vi "AH Bridge Read.vi"(6 "Read Frequency":bool, 9 "Boolean":bool, 10 "Average Time (mS)":u32, 11 "Instrument Address":refnum<visa-resource-name>) -> (2 "Measurement":dbl[](array[numeric]) format="%_6e", 3 "dup Instrument Address":refnum<visa-resource-name>)   [LabVIEW 2021]
uses:
  <vilib>/regexp/Match Regular Expression.xnode
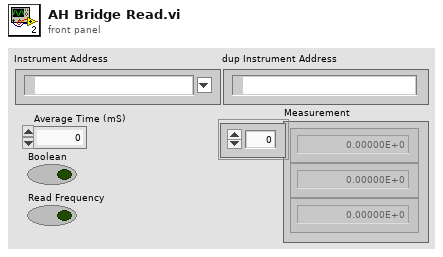
[diagram p1: front panel]
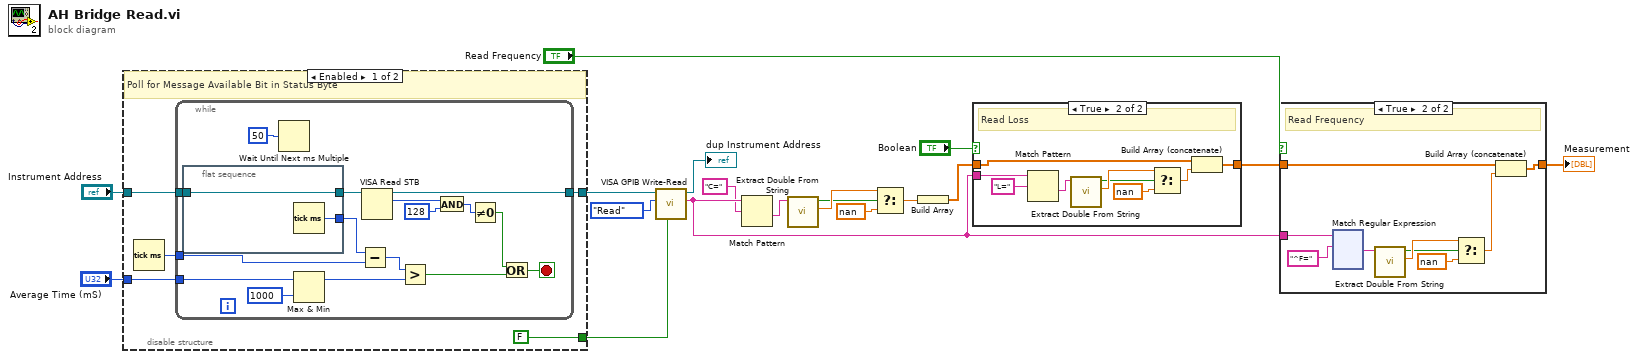
[diagram p0: block diagram]
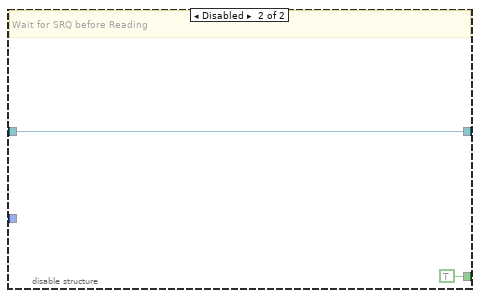
[diagram p2: hidden frame]
diagram:
  n1 = disable-structure shown="Enabled" {
    disable-tunnel: [w23 w43] -> w17
    disable-tunnel: "Instrument Address" -> [w21 w43]
    disable-tunnel: "Average Time (mS)" -> [w20 _]
    disable-tunnel: [FALSE ("Wait For SRQ") TRUE ("Wait For SRQ")] -> w3
    frame Enabled {
      # "Poll for Message Available Bit in Status Byte"
      n2 = Tick Count (ms)() -> (millisecond timer value=w22:u32)
      n3 = while {
        tunnel: [w33] -> w23
        tunnel: w21 -> [w29]
        tunnel: w22 -> [w32]
        tunnel: w20 -> [w27]
        stop <- w38 stop-if-true
        n4 = flat-sequence {
          tunnel: [w41] -> w31
          tunnel: [w40] -> w28
          tunnel: w29 -> [w40]
          frame #0 {
            n5 = Tick Count (ms)() -> (millisecond timer value=w41:u32)
          }
        }
        n6 = Wait Until Next ms Multiple(millisecond multiple=u32 50) -> ()  [unwired: 1 out]
        n7 = Max & Min(x=w27, y=u32 1000) -> (max(x,y)=w26:u32)  [unwired: 1 out]
        n8 = Subtract(x=w31, y=w32) -> (x-y=w30:u32)
        n9 = VISA Read STB(11:w28) -> (2:w34:u16, 3:w33:refnum<visa-resource-name>)  [unwired: 1 in, 1 out]
        n10 = Greater?(x=w30, y=w26) -> (0:w37:bool)
        n11 = And(x=w34, y=u16 128) -> (x .and. y?=w35:u16)
        n12 = Not Equal To 0?(x=w35) -> (x != 0?=w36:bool)
        n13 = Or(x=w36, y=w37) -> (x .or. y?=w38:bool)
      }
    }
    frame Disabled {
      # "Wait for SRQ before Reading"
    }
  }
  n14 = call "VISA GPIB Write-Read.vi"("Wait For SRQ"=w3, "Action"=enum16{"Write", "Read", "Write & Read"}."Read", "VISA resource name"=w17) -> ("String Returned"=w13:string, "dup VISA Session"=→"dup Instrument Address":refnum<visa-resource-name>)  [unwired: 5 in, 2 out]
  n15 = Match Pattern(string=w13, regular expression="C=") -> (after substring=w7:string)  [unwired: 1 in, 3 out]
  n16 = call "Extract Double From String.vi"("string"=w7) -> ("floating pt. number"=w9:dbl, "valid"=w8:bool)  [unwired: 3 in, 2 out]
  n17 = Select(t=w9, s=w8, f=nan) -> (s? t:f=w11:dbl)
  n18 = Build Array(w11) -> (w14:dbl[])
  n19 = case shown="True" "Boolean" {
    tunnel: w13 -> [_ w51]
    tunnel: w14 -> [w44 w46]
    tunnel: [w44 w45] -> w15
    frame False {
    }
    frame True {
      # "Read Loss"
      n20 = Match Pattern(string=w51, regular expression="L=") -> (after substring=w52:string)  [unwired: 1 in, 3 out]
      n21 = call "Extract Double From String.vi"("string"=w52) -> ("floating pt. number"=w49:dbl, "valid"=w48:bool)  [unwired: 3 in, 2 out]
      n22 = Select(t=w49, s=w48, f=nan) -> (s? t:f=w47:dbl)
      n23 = Build Array (concatenate)(w46, w47) -> (w45:dbl[])
    }
  }
  n24 = case shown="True" "Read Frequency" {
    tunnel: w13 -> [_ w55]
    tunnel: w15 -> [w54 w57]
    tunnel: [w54 w56] -> w16
    frame False {
    }
    frame True {
      # "Read Frequency"
      n25 = xnode "Match Regular Expression"("input string"=w55, "regular expression"="^F=") -> ("after match"=w62:string)  [unwired: 4 in, 4 out]
      n26 = call "Extract Double From String.vi"("string"=w62) -> ("floating pt. number"=w60:dbl, "valid"=w59:bool)  [unwired: 3 in, 2 out]
      n27 = Select(t=w60, s=w59, f=nan) -> (s? t:f=w58:dbl)
      n28 = Build Array (concatenate)(w57, w58) -> (w56:dbl[])
    }
  }
  "Measurement" <- w16
